vi "Get VI Ref.vi"(8 "error in":errorcluster, 9 "Name.vi":string, 10 "Owned Items[]":refnum<vi>[](array[refnum])) -> (0 "error out":errorcluster, 1 "VI Reference":refnum<vi>)   [LabVIEW 2020, in "_Rename.lvlib" / "_Rename.lvclass"]
uses:
  _Rename.lvclass
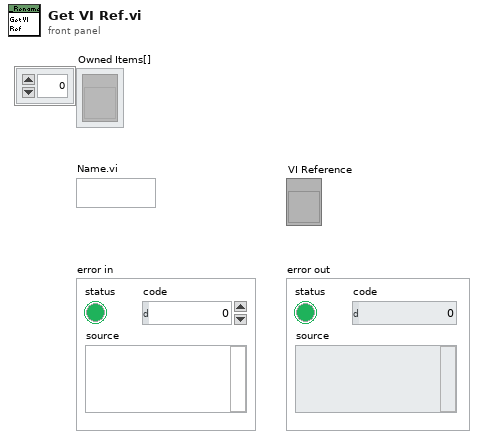
[diagram p1: front panel]
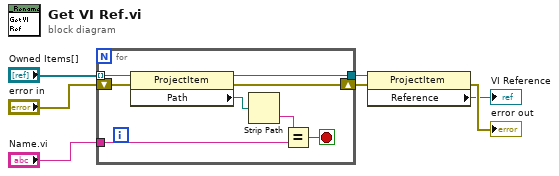
[diagram p0: block diagram]
diagram:
  n1 = for {
    tunnel: "Owned Items[]" -> [w15] mode=indexing
    shift-right: [w13] -> w6
    shift-left: "error in" -> [w14]
    tunnel: [w12] -> w7
    tunnel: "Name.vi" -> [w8]
    stop <- w11 stop-if-true
    n2 = property class="ProjectItem"(reference=w15, error in=w14) -> (reference out=w12:refnum<vi>, error out=w13:errorcluster, "Path"=w10:path)
    n3 = Strip Path(path=w10) -> (name=w9:string)  [unwired: 1 out]
    n4 = Equal?(x=w9, y=w8) -> (x = y?=w11:bool)
  }
  n5 = property class="ProjectItem"(reference=w7, error in=w6) -> (error out=→"error out":errorcluster, "Reference"=→"VI Reference":refnum<vi>)  [unwired: 1 out]
